vi "ImageRotationReflexion.vi"() -> ()   [LabVIEW 2011]
uses:
  <vilib>/gmath/interp.llb/Interpolate 2D (2d X,Y).vi
  <vilib>/gmath/NI_Gmath.lvlib
panel:
  out "Total Size":i32
  out "Y":i32[](array[numeric])
  out "X":i32[](array[numeric])
  out "Z":dbl[](array[numeric])
  out "ImgArray OUT":u32[][](graph)
  in  "ImgArray IN":u32[][](graph)=array640x480[307200 elements]
  out "Array OUT":dbl[][](array[numeric])
  in  "Array IN":dbl[][](array[numeric])
  in  "Angle [°]":dbl(knob) scale=-90.0..90.0
  in  "Invert Y":bool
  in  "Invert X":bool
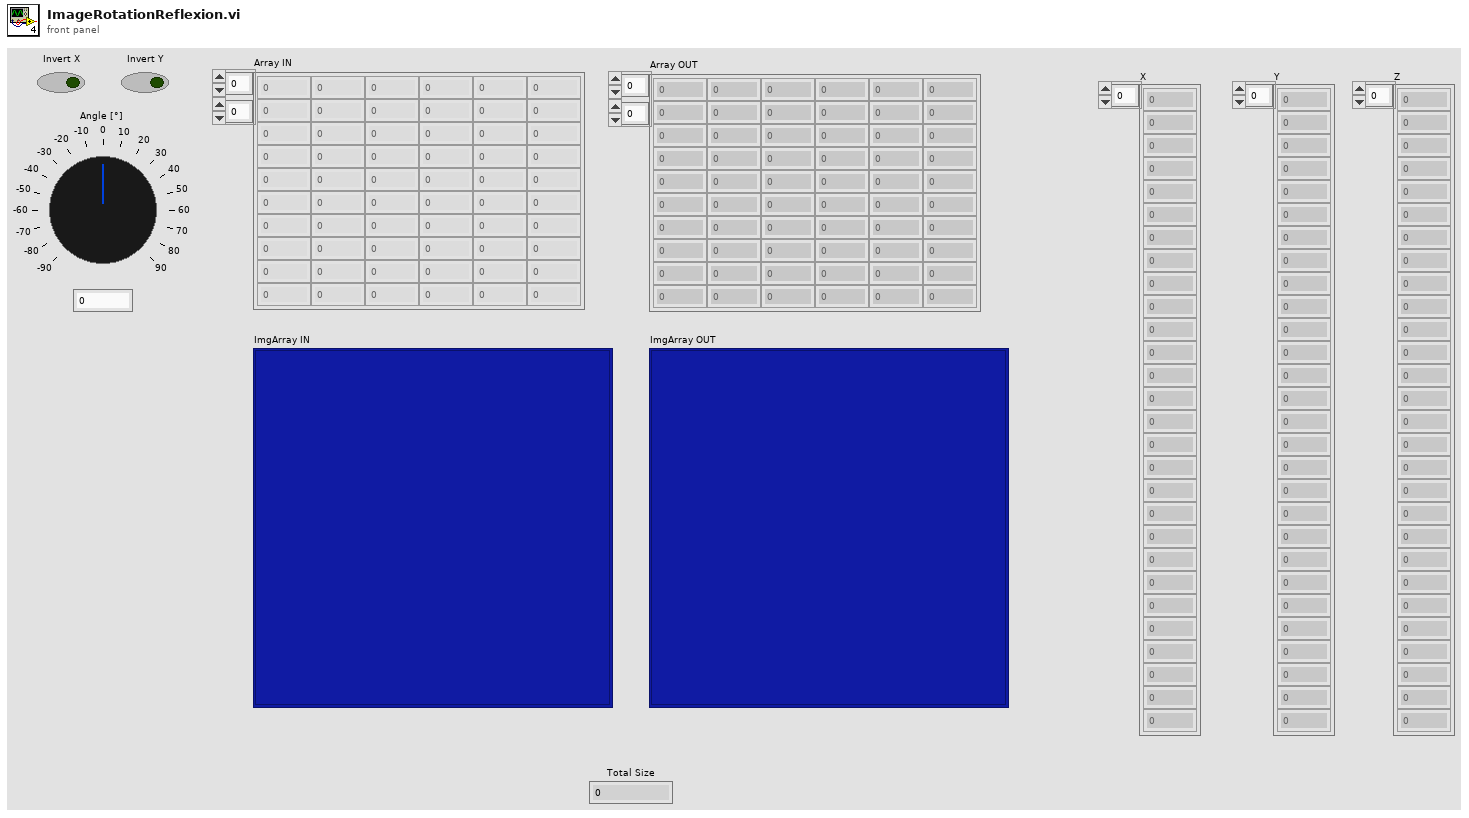
[diagram p1: front panel]
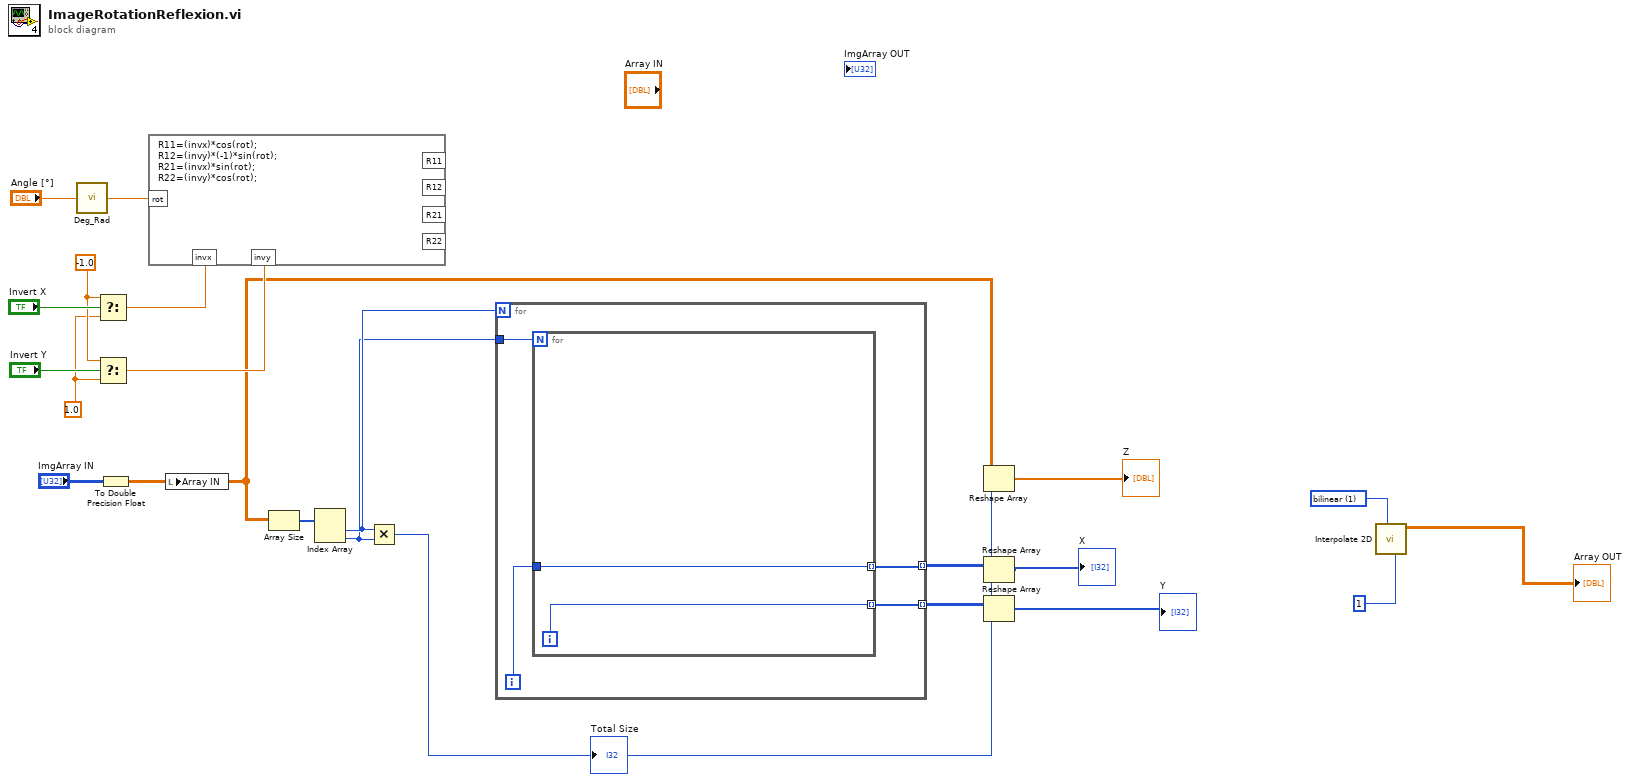
[diagram p0: block diagram]
diagram:
  w12 = 1.0 ("t")
  w13 = -1.0 ("t")
  w22 = 1 items=["nearest", "bilinear", "bicubic", "bicubic spline"] ("method")
  n1 = call "Deg_Rad.vi"("Angle"="Angle [°]") -> ("RadRot"=w18:dbl)
  n2 = Select(t=w13, s="Invert X", f=w12) -> (s? t:f=w15:dbl)
  n3 = Select(t=w13, s="Invert Y", f=w12) -> (s? t:f=w14:dbl)
  n4 = To Double Precision Float(number="ImgArray IN") -> (double precision float=w4:dbl[][])
  n5 = formula code="R11=(invx)*cos(rot);\nR12=(invy)*(-1)*sin(rot);\nR21=(invx)*sin(rot);\nR22=(invy)*cos(rot);"("rot"=w18, "invx"=w15, "invy"=w14) -> ()  [unwired: 4 out]
  n6 = local write "Array IN"(w4) -> ()
  n7 = Array Size(array=w4) -> (size(s)=w10:i32[])
  n8 = Index Array(array=w10) -> (element #1=w9:i32, element #2=w8:i32)  [unwired: 2 in]
  n9 = Multiply(x=w9, y=w8) -> (x*y=w3:i32)
  "Total Size" <- w3
  n10 = for {
    N: w9 -> [_]
    tunnel: w8 -> [w25]
    tunnel: [w24] -> w6 mode=indexing
    tunnel: [w23] -> w7 mode=indexing
    i -> [w26]
    n11 = for {
      N: w25 -> [_]
      tunnel: w26 -> [w28]
      tunnel: [w28] -> w24 mode=indexing
      tunnel: [w27] -> w23 mode=indexing
      i -> [w27]
    }
  }
  n12 = Reshape Array(w4, w3) -> (→"Z":dbl[])
  n13 = Reshape Array(w6, w3) -> (→"X":i32[])
  n14 = Reshape Array(w7, w3) -> (→"Y":i32[])
  n15 = call-poly <vilib>:"Interpolate 2D.vi"("ntimes"=1, "method"=w22) -> ("zi"=→"Array OUT":dbl[][])  [unwired: 6 in, 3 out]
